vi "Timing Status Size.vi"(8 "error in (no error)":errorcluster) -> (0 "error out":errorcluster, 3 "size":u64 format="%d bytes")   [LabVIEW 2019, in "DSF Core.lvlib" / "Timing Status Pointer.lvclass"]
uses:
  Timing Status Pointer.lvclass
  Timing Status Data.ctl
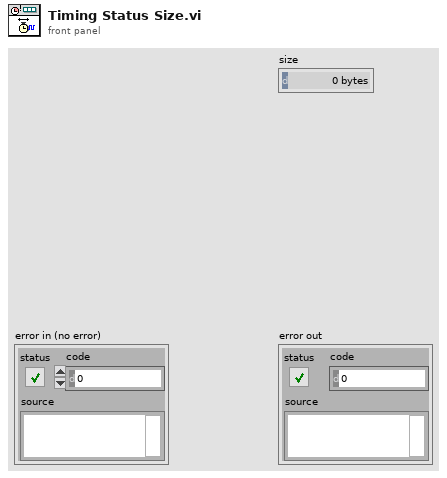
[diagram p1: front panel]
types:
  T1 = typedef "DSF Core.lvlib/Timing Status Pointer.lvclass/Timing Status Data.ctl" = cluster{"rx start time":u32, "rx end time":u32, "tx start time":u32, "tx end time":u32, "cycle start time":u32, "cycle end time":u32, "prev start time":u32}
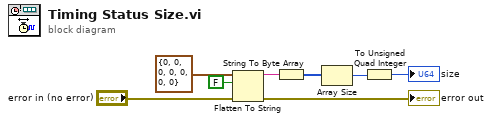
[diagram p0: block diagram]
diagram:
  n1 = Flatten To String(anything=T1 {"rx start time"=0, "rx end time"=0, "tx start time"=0, "tx end time"=0, "cycle start time"=0, "cycle end time"=0, "prev start time"=0} ("Transfer Group status"), prepend array or string size? (T)=FALSE, error in (no error)="error in (no error)") -> (data string=w7:string, error out=→"error out":errorcluster)  [unwired: 1 in, 1 out]
  n2 = String To Byte Array(string=w7) -> (unsigned byte array=w6:u8[])
  n3 = Array Size(array=w6) -> (size(s)=w5:i32)
  n4 = To Unsigned Quad Integer(1:w5) -> (0:→"size":u64)
